vi "EXFO 3150 Variable Attenuator.vi"() -> ()   [LabVIEW 2018]
doc: "This example will show how to create simple instrument drivers high level example for EXFO IQS 3150 instrument performing initialization, action(s) and close activity.\n\nIt sets the wavelength, control mode, input attenuation values of the instrument and queries the value for Input Attenuation."
uses:
  <vilib>/Utility/error.llb/DialogType.ctl
  3150.lvlib
panel:
  in  "Attenuation Type (0:Current)":u16(ring) items=["Current", "MINimum", "MAXimum", "DEFault"]
  out "Input Attenuation":dbl format="%#_6e"
  out "error out":errorcluster
  in  "User Defined Attenuation Value (5.0000)":dbl=5.0 format="%_5g"
  in  "User Defined Wavelength Value (1310)":dbl=1310.0
  in  "Platform Slot Number (10)":i16=10 min=-1 max=255
  in  "Input Attenuation (0:MINimum)":i32(ring) items=["MINimum", "MAXimum", "DEFault", "User Defined Value"]
  in  "Control Mode (0:ATTenuation)":u16(ring) items=["ATTenuation", "POWer"]
  in  "Wavelength Unit (0:NM)":u16(ring) items=["NM", "M"]
  in  "Wavelength (0:MINimum)":i32(ring) items=["MINimum", "MAXimum", "DEFault", "User Defined Value"]
  in  "VISA resource name":refnum<visa-resource-name>
  # "(c) 2010 EXFO Inc. ALL RIGHTS RESERVED."
  # "Trigger Controls"
  # "Instrument Readings"
  # "Set the input wavelength for the instrument"
  # "Returns the output power, in dBM"
  # "Select the wavelength unit"
  # "Set the attenuation control mode."
  # "Set the input attenuation value for the instrument"
  # "Selects the token for information retrievel"
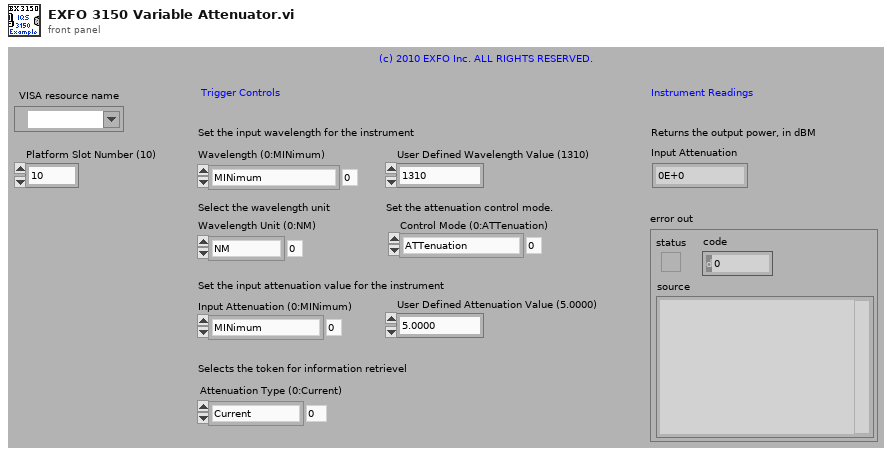
[diagram p1: front panel]
types:
  T1 = typedef "DialogType.ctl" = u16
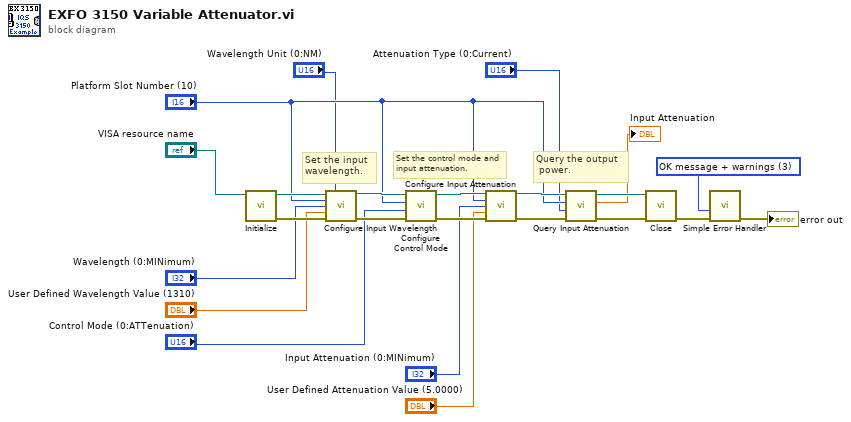
[diagram p0: block diagram]
diagram:
  w8 = T1 3 items=["no dialog", "OK message", "continue or stop message", "OK message + warnings", "continue/stop + warnings"] ("type of dialog (OK msg:1)")
  # "Query the output\n power."
  # "Set the control mode and input attenuation."
  # "Set the input \nwavelength."
  n1 = call "Initialize.vi"("VISA resource name"="VISA resource name") -> ("error out"=w20:errorcluster, "VISA resource name out"=w21:refnum<visa-resource-name>)  [unwired: 1 in, 8 out]
  n2 = call "Configure Input Wavelength.vi"("VISA resource name"=w21, "Wavelength Unit (0:NM)"="Wavelength Unit (0:NM)", "Platform Slot Number (10)"="Platform Slot Number (10)", "Wavelength (0:MINimum)"="Wavelength (0:MINimum)", "User Defined Wavelength Value (1310)"="User Defined Wavelength Value (1310)", "error in (no error)"=w20) -> ("VISA resource name out"=w19:refnum<visa-resource-name>, "error out"=w18:errorcluster)  [unwired: 8 out]
  n3 = call "Configure Control Mode.vi"("error in (no error)"=w18, "Control Mode (0:ATTenuation)"="Control Mode (0:ATTenuation)", "Platform Slot Number (10)"="Platform Slot Number (10)", "VISA resource name"=w19) -> ("error out"=w16:errorcluster, "VISA resource name out"=w17:refnum<visa-resource-name>)  [unwired: 6 out]
  n4 = call "Configure Input Attenuation.vi"("VISA resource name"=w17, "Platform Slot Number (10)"="Platform Slot Number (10)", "Input Attenuation (0:MINimum)"="Input Attenuation (0:MINimum)", "User Defined Attenuation Value (5.0000)"="User Defined Attenuation Value (5.0000)", "error in (no error)"=w16) -> ("VISA resource name out"=w15:refnum<visa-resource-name>, "error out"=w14:errorcluster)  [unwired: 9 out]
  n5 = call "Query Input Attenuation.vi"("error in (no error)"=w14, "Attenuation Type (0:Current)"="Attenuation Type (0:Current)", "Platform Slot Number (10)"="Platform Slot Number (10)", "VISA resource name"=w15) -> ("error out"=w13:errorcluster, "Input Attenuation"=→"Input Attenuation":dbl, "VISA resource name out"=w12:refnum<visa-resource-name>)  [unwired: 5 out]
  n6 = call "Close.vi"("error in (no error)"=w13, "VISA resource name"=w12) -> ("error out"=w9:errorcluster)  [unwired: 9 out]
  "error out" <- w9
  n7 = call <vilib>:"Simple Error Handler.vi"("type of dialog (OK msg:1)"=w8, "error in (no error)"=w9) -> ()  [unwired: 8 out]
